vi "SD Read Value.vi"   [LabVIEW 2017]
doc: "A polyVI that will read the SmartDashboard entry -- /prefix/name. Use the poly selector to choose the type to read."
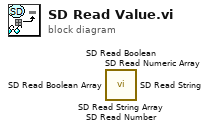
[diagram p0: block diagram]
diagram:
  n1 = call <vilib>:"SD Read String Array.vi"() -> ()  [unwired: 10 in, 2 out]
  n2 = call <vilib>:"SD Read Numeric Array.vi"() -> ()  [unwired: 9 in, 3 out]
  n3 = call <vilib>:"SD Read Boolean Array.vi"() -> ()  [unwired: 9 in, 3 out]
  n4 = call <vilib>:"SD Read String.vi"() -> ()  [unwired: 9 in, 3 out]
  n5 = call <vilib>:"SD Read Number.vi"() -> ()  [unwired: 9 in, 3 out]
  n6 = call <vilib>:"SD Read Boolean.vi"() -> ()  [unwired: 9 in, 3 out]
